vi "SetAutoapproachDetails.vi"(0 "AA Details Cluster":T1={"Axis"=0, "Direction"=-2147483648, "Device"=-2147483648, "Trigger Pol."=-2147483648, "Hold Time [us]"=-2147483648, "GND while Approach"=-2147483648} {"GND while Approach" items=["[read only]"=-2147483648, "No"=0, "Yes"=1]; "Trigger Pol." items=["[read only]"=-2147483648, "high active"=0, "low active"=1]; "Device" items=["[read only]"=-2147483648, "ANC300"=0, "TTL via DAC2"=1, "LVTTL via DAC2"=2, "ANC350 via NSL A"=3, "ANC350 via NSL B"=4, "attoSTM NSL A"=5, "attoSTM NSL B"=6]; "Direction" items=["[read only]"=-2147483648, "forward"=0, "backward"=1]; "Axis" items=["[read only]"=-2147483648, "Axis 1"=0, "Axis 2"=1, "Axis 3"=2]}, 5 "error in":T7) -> (14 "Output Cluster":T1={"Axis"=0, "Direction"=-2147483648, "Device"=-2147483648, "Trigger Pol."=-2147483648, "Hold Time [us]"=-2147483648, "GND while Approach"=-2147483648} {"GND while Approach" items=["[read only]"=-2147483648, "No"=0, "Yes"=1]; "Trigger Pol." items=["[read only]"=-2147483648, "high active"=0, "low active"=1]; "Device" items=["[read only]"=-2147483648, "ANC300"=0, "TTL via DAC2"=1, "LVTTL via DAC2"=2, "ANC350 via NSL A"=3, "ANC350 via NSL B"=4, "attoSTM NSL A"=5, "attoSTM NSL B"=6]; "Direction" items=["[read only]"=-2147483648, "forward"=0, "backward"=1]; "Axis" items=["[read only]"=-2147483648, "Axis 1"=0, "Axis 2"=1, "Axis 3"=2]}, 19 "error out":T7)   [LabVIEW 2016]
doc: "Sets up some additional and more special parameters for the auto approach mode. The cluster contains:\n\n- Axis (integer) [0 -- Axis 1; 1 -- Axis 2; 2 -- Axis 3]\n- Direction (integer) [0 -- forward; 1 -- backward]\n- Device (integer) [0 -- ANC150; 1 -- TTL via DAC2; 2 -- LVTTL via DAC2]\n- Trigger Pol. (integer) [0 -- high active; 1 -- low active]\n- Hold Time in us (integer) [0 to 300000]\n- GND while Approach (integer) [0 -- no; 1 -- yes]\nBy passing -Inf (float) or -2147483648 (integer) as input values, the corresponding parameter(s) will be read out."
uses:
  Controls/Autoapproach-Details_Parameters.ctl
  Controls/Autoapproach-Axis_Selection.ctl
  Controls/Appraoch-Direction_Selection.ctl
  Controls/Autoapproach-Device_Selection.ctl
  Controls/Autoapproach-Trigger_Selection.ctl
  Controls/Ground-while-Appraoch_Selection.ctl
  Controls/Error_Out.ctl
  Files_ASC500/DLL/ASC500_RemoteControlV27.dll
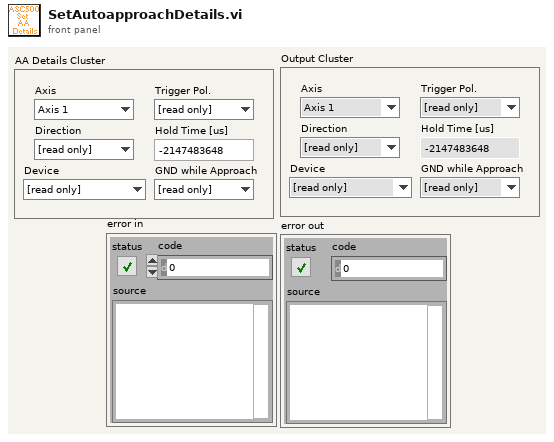
[diagram p1: front panel]
types:
  T1 = typedef "Autoapproach-Details_Parameters.ctl" = cluster{"Axis":T2, "Direction":T3, "Device":T4, "Trigger Pol.":T5, "Hold Time [us]":i32, "GND while Approach":T6}
  T2 = typedef "Autoapproach-Axis_Selection.ctl" = i32
  T3 = typedef "Appraoch-Direction_Selection.ctl" = i32
  T4 = typedef "Autoapproach-Device_Selection.ctl" = i32
  T5 = typedef "Autoapproach-Trigger_Selection.ctl" = i32
  T6 = typedef "Ground-while-Appraoch_Selection.ctl" = i32
  T7 = typedef "Error_Out.ctl" = errorcluster
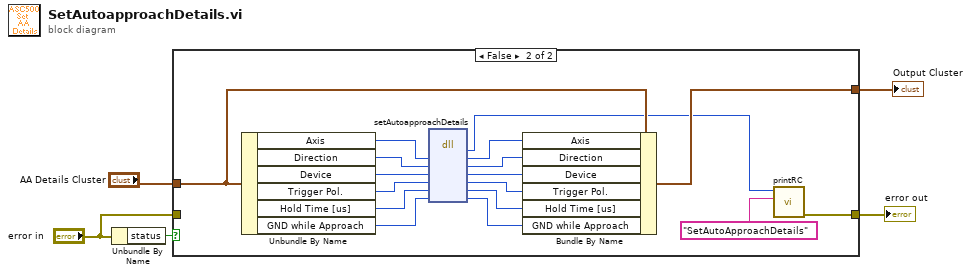
[diagram p0: block diagram]
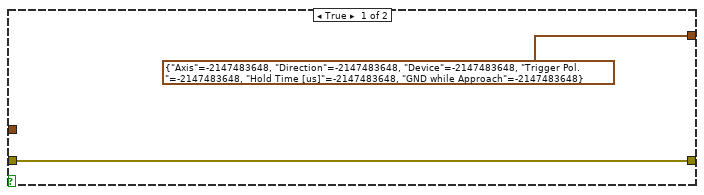
[diagram p2: hidden frame]
diagram:
  n1 = Unbundle By Name("error in") -> ("status"=w5:bool)
  n2 = case shown="False" w5 {
    tunnel: [w6 w10] -> w4
    tunnel: "AA Details Cluster" -> [_ w15]
    tunnel: [T1 {"Axis"=-2147483648, "Direction"=-2147483648, "Device"=-2147483648, "Trigger Pol."=-2147483648, "Hold Time [us]"=-2147483648, "GND while Approach"=-2147483648} ("Autoapproach Details Cluster") w14] -> w2
    tunnel: "error in" -> [w6 _]
    frame True {
    }
    frame False {
      n3 = Unbundle By Name(w15) -> ("Axis"=w21:T2, "Direction"=w22:T3, "Device"=w13:T4, "Trigger Pol."=w12:T5, "Hold Time [us]"=w23:i32, "GND while Approach"=w24:T6)
      n4 = dll-call lib="G:/SCMOperations/Share/ELE/Produkt Information/ASC500/04 Remote Control/02 development versions/2018Nov06/Files_ASC500/DLL/ASC500_RemoteControlV27.dll" fn="setAutoapproachDetails"("Axis"=w21, "Direction"=w22, "Device"=w13, "Trigger Pol."=w12, "Hold Time"=w23, "GND while Approach"=w24) -> ("return type"=w9:i32, "Axis"=w20:i32, "Direction"=w19:i32, "Device"=w11:i32, "Trigger Pol."=w18:i32, "Hold Time"=w17:i32, "GND while Approach"=w16:i32)  [unwired: 3 in, 2 out]
      n5 = Bundle By Name(cluster=w15, "Axis"=w20, "Direction"=w19, "Device"=w11, "Trigger Pol."=w18, "Hold Time [us]"=w17, "GND while Approach"=w16) -> (w14:T1)
      n6 = call "printRC.vi"("additional information"="SetAutoApproachDetails", "RC"=w9) -> ("error out"=w10:T7)  [unwired: 9 in]
    }
  }
  "error out" <- w4
  "Output Cluster" <- w2
